vi "Database.GetThisStatus.vi"(8 "error in":errorcluster, 9 "Serial":string, 10 "Variant":string, 11 "Data in":T1) -> (0 "error out":errorcluster, 3 "Data out":T1)   [LabVIEW 2016]
uses:
  Database.Data.ctl
  Database.Data.Sets.ctl
  Handler/Database.Handler.Data.Status.ctl
  Database.Gui.ctl
  Database.Gui.SingleTestValue.ctl
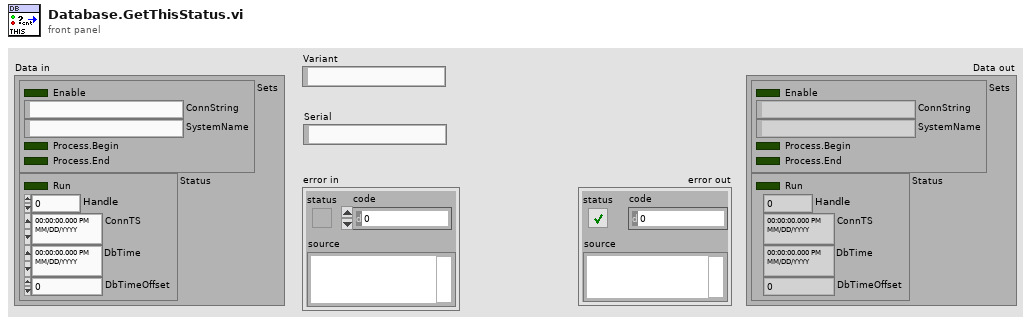
[diagram p1: front panel]
types:
  T1 = typedef "Database.Data.ctl" = cluster{"Sets":T2, "Status":T3}
  T2 = typedef "Database.Data.Sets.ctl" = cluster{"Enable":bool, "ConnString":string, "SystemName":string, "Process.Begin":bool, "Process.End":bool}
  T3 = typedef "Database.Handler.Data.Status.ctl" = cluster{"Run":bool, "Handle":i32, "ConnTS":timestamp, "DbTime":timestamp, "DbTimeOffset":dbl}
  T4 = typedef "Database.Gui.ctl" = cluster{"Station":string, "ButtonEnabled":bool, "Values":T5[]}
  T5 = typedef "Database.Gui.SingleTestValue.ctl" = cluster{"EV_name":string, "Value":dbl, "LimitL":dbl, "LimitH":dbl, "Status":u8}
  T6 = typedef "ProdaNG.Identification.ctl" = cluster{"processId":i32, "systemId":i32, "processStepId":i32, "wabcoPartId":i32}
  T7 = typedef "ProdaNG.Product.ctl" = cluster{"c_id":string, "wabcoPartId":i32, "serialNumber":string, "comment":string, "individual":i32, "crProcessStepId":i32, "mdProcessStepId":i32, "crTime":string, "mdTime":string}
  T8 = typedef "ProdaNG.TestStep.ctl" = cluster{"i_id":i32, "processStepId":i32, "testSequence":i32, "testOrder":i32, "mdReason":string, "mdUser":string, "mdTime":string, "description":string}
  T9 = typedef "ProdaNG.TestValue.ctl" = cluster{"i_id":i32, "testStepId":i32, "releaseId":i32, "unitId":i32, "contentId":string, "previewId":string, "maximum":dbl, "minimum":dbl, "valueText":string, "testValueSequence":i32, "history":i32, "mdReason":string, "mdUser":string, "mdTime":string, "description":string}
  T10 = typedef "ProdaNG.ProcessResult.ctl" = cluster{"c_id":string, "productId":string, "processId":i32, "statusId":i32, "startTime":string, "endTime":string}
  T11 = typedef "ProdaNG.ProcessStepResult.ctl" = cluster{"c_id":string, "processResultId":string, "processStepId":i32, "statusId":i32, "operatorId":i32, "startTime":string, "endTime":string}
  T12 = typedef "ProdaNG.TestStepResult.ctl" = cluster{"c_id":string, "processStepResultId":string, "testStepId":i32, "statusId":i32}
  T13 = typedef "ProdaNG.TestValueResult.ctl" = cluster{"c_id":string, "testStepResultId":string, "testValueId":i32, "result":dbl, "statusId":i32, "contentId":string}
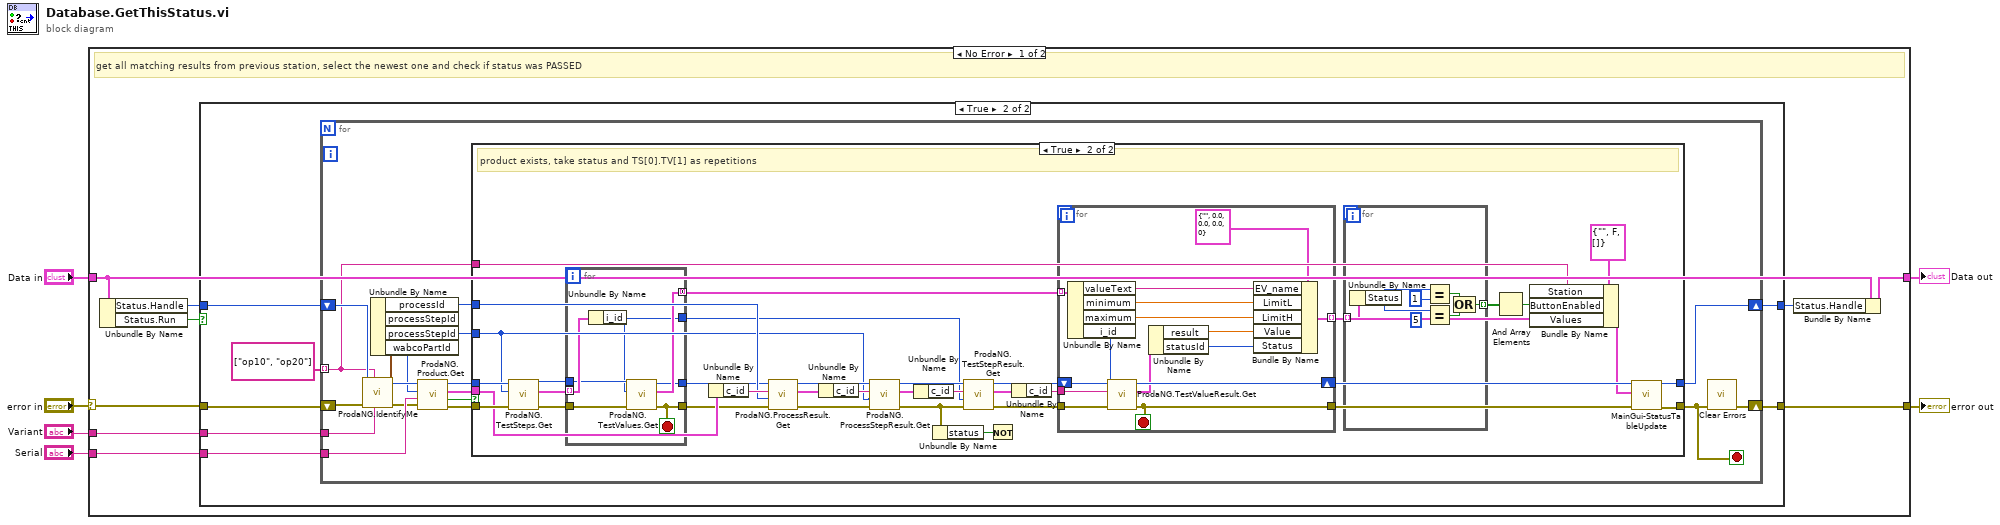
[diagram p0: block diagram]
diagram:
  n1 = case shown="No Error" "error in" {
    selector: "error in" -> [w14 w110]
    tunnel: [w15 w110] -> w6
    tunnel: "Data in" -> [w12 w109]
    tunnel: [w11 w109] -> w3
    tunnel: "Serial" -> [w8 _]
    tunnel: "Variant" -> [w7 _]
    frame No Error {
      # "get all matching results from previous station, select the newest one and check if status was PASSED"
      n2 = Unbundle By Name(w12) -> ("Status.Handle"=w13:i32, "Status.Run"=w9:bool)
      n3 = case shown="True" w9 {
        tunnel: w14 -> [w16 w21]
        tunnel: [w16 w18] -> w15
        tunnel: w13 -> [w17 w23]
        tunnel: [w17 w24] -> w10
        tunnel: w8 -> [_ w22]
        tunnel: w7 -> [_ w19]
        frame False {
        }
        frame True {
          n4 = for {
            tunnel: w22 -> [w36]
            shift-right: [w42] -> w18
            shift-left: w21 -> [w35]
            shift-right: [w37] -> w24
            shift-left: w23 -> [w34]
            tunnel: string[] ["op10", "op20"] -> [w27] mode=indexing
            tunnel: w19 -> [w26]
            stop <- w25 stop-if-true
            n5 = call "ProdaNG.IdentifyMe.vi"("wabcoNumber"=w26, "systemName"=w27, "error in"=w35, "dbHandleIn"=w34) -> ("error out"=w31:errorcluster, "Identification"=w32:T6, "dbHandle"=w33:i32)  [unwired: 5 in]
            n6 = Unbundle By Name(w32) -> ("processId"=w29:i32, "processStepId"=w28:i32, "wabcoPartId"=w30:i32)  [unwired: 1 out]
            n7 = call "ProdaNG.Product.Get.vi"("error in (no error)"=w31, "serialNumber"=w36, "wabcoPartId"=w30, "dbHandle"=w33) -> ("error out"=w40:errorcluster, "found"=w38:bool, "Product"=w39:T7, "dbHandle out"=w41:i32)  [unwired: 4 in]
            n8 = case shown="True" w38 {
              tunnel: w40 -> [w44 w63]
              tunnel: [w44 w48] -> w25
              tunnel: w41 -> [w43 w62]
              tunnel: w39 -> [_ w61]
              tunnel: [w43 w67] -> w37
              tunnel: w29 -> [_ w64]
              tunnel: w28 -> [_ w45]
              tunnel: w27 -> [_ w52]
              frame False {
                # "product missing"
              }
              frame True {
                # "product exists, take status and TS[0].TV[1] as repetitions"
                n9 = call "ProdaNG.TestSteps.Get.vi"("error in (no error)"=w63, "processStepId"=w45, "dbHandleIn"=w62) -> ("error out"=w58:errorcluster, "TestSteps"=w60:T8[], "dbHandle"=w59:i32)  [unwired: 6 in]
                n10 = for {
                  tunnel: w60 -> [w108] mode=indexing
                  tunnel: w59 -> [w105]
                  tunnel: w58 -> [w107]
                  tunnel: [w106] -> w55 mode=concatenating
                  tunnel: [w104] -> w57
                  tunnel: [w103] -> w56
                  tunnel: [w102] -> w46
                  stop <- w104 stop-if-true
                  n11 = Unbundle By Name(w108) -> ("i_id"=w102:i32)
                  n12 = call "ProdaNG.TestValues.Get.vi"("error in (no error)"=w107, "testStepId"=w102, "dbHandleIn"=w105) -> ("error out"=w104:errorcluster, "TestStepValues"=w106:T9[], "dbHandle"=w103:i32)  [unwired: 6 in]
                }
                n13 = Unbundle By Name(w61) -> ("c_id"=w75:string)
                n14 = call "ProdaNG.ProcessResult.Get.vi"("error in (no error)"=w57, "processId"=w64, "productId"=w75, "dbHandle"=w56) -> ("error out"=w77:errorcluster, "ProcessResult"=w79:T10, "dbHandle out"=w78:i32)  [unwired: 4 in, 1 out]
                n15 = Unbundle By Name(w79) -> ("c_id"=w76:string)
                n16 = call "ProdaNG.ProcessStepResult.Get.vi"("error in (no error)"=w77, "processStepId"=w45, "processResultId"=w76, "dbHandle"=w78) -> ("error out"=w66:errorcluster, "ProcessStepResult"=w72:T11, "dbHandle out"=w73:i32)  [unwired: 4 in, 1 out]
                n17 = Unbundle By Name(w72) -> ("c_id"=w71:string)
                n18 = Unbundle By Name(w66) -> ("status"=w65:bool)
                n19 = call "ProdaNG.TestStepResult.Get.vi"("error in (no error)"=w66, "testStepId"=w46, "processStepResulttId"=w71, "dbHandle"=w73) -> ("error out"=w69:errorcluster, "TestStepResult"=w74:T12, "dbHandle out"=w70:i32)  [unwired: 4 in, 1 out]
                n20 = Not(x=w65) -> ()  [unwired: 1 out]
                n21 = Unbundle By Name(w74) -> ("c_id"=w68:string)
                n22 = for {
                  tunnel: w68 -> [w99]
                  shift-right: [w98] -> w67
                  shift-left: w70 -> [w101]
                  tunnel: w69 -> [w100]
                  tunnel: [w97] -> w49
                  tunnel: w55 -> [w96] mode=indexing
                  tunnel: [w87] -> w50 mode=indexing
                  stop <- w97 stop-if-true
                  n23 = Unbundle By Name(w96) -> ("valueText"=w92:string, "minimum"=w91:dbl, "maximum"=w90:dbl, "i_id"=w95:i32)
                  n24 = call "ProdaNG.TestValueResult.Get.vi"("error in (no error)"=w100, "testValueId"=w95, "testStepResultId"=w99, "dbHandle"=w101) -> ("error out"=w97:errorcluster, "TestValueResult"=w94:T13, "dbHandle"=w98:i32)  [unwired: 5 in]
                  n25 = Unbundle By Name(w94) -> ("result"=w89:dbl, "statusId"=w88:i32)
                  n26 = Bundle By Name(cluster=T5 {"EV_name"="", "Value"=0.0, "LimitL"=0.0, "LimitH"=0.0, "Status"=0} ("Cluster"), "EV_name"=w92, "LimitL"=w91, "LimitH"=w90, "Value"=w89, "Status"=w88) -> (w87:T5)
                }
                n27 = for {
                  tunnel: w50 -> [w80] mode=indexing
                  tunnel: [w81] -> w54 mode=indexing
                  n28 = Unbundle By Name(w80) -> ("Status"=w86:u8)
                  n29 = Equal?(x=w86, y=u8 1) -> (x = y?=w83:bool)
                  n30 = Equal?(x=w86, y=u8 5) -> (x = y?=w82:bool)
                  n31 = Compound Arithmetic op=OR(w83, w82) -> (w81:bool)
                }
                n32 = And Array Elements(Boolean array=w54) -> (logical AND=w51:bool)
                n33 = Bundle By Name(cluster=T4 {"Station"="", "ButtonEnabled"=FALSE, "Values"=[]} ("TestValueResult"), "Station"=w52, "ButtonEnabled"=w51, "Values"=w50) -> (w47:T4)
                n34 = call "MainGui-StatusTableUpdate.vi"("error in (no error)"=w49, "TestValueResult"=w47) -> ("error out"=w48:errorcluster)  [unwired: 9 in]
              }
            }
            n35 = call <vilib>:"Clear Errors.vi"("error in (no error)"=w25) -> ("error out"=w42:errorcluster)  [unwired: 5 in, 1 out]
          }
        }
      }
      n36 = Bundle By Name(cluster=w12, "Status.Handle"=w10) -> (w11:T1)
    }
    frame Error {
    }
  }
  "error out" <- w6
  "Data out" <- w3
